vi "Stimulus.Create.vi"(8 "error in (no error)":errorcluster, 11 "State Variables":T1={"Events.State"=refnum, "Events.Test Result"=refnum, "Events.Progress"=refnum, "INI.Settings"={"Build Location"=path "C:/Simple Sequence Editor/SequenceRepo", "LoggingLocation"=path "", "Sequence.AbortChannel"="", "Sequence.IterationInfoChannel"="", "Sequence.DurationChannel"="", "Sequence.StepInfoChannel"="", "Sequence.SkipChannel"="", "PlotChannels"=[], "Sequence.InitializeScript"=path "C:/Simple Sequence Editor/SequenceRepo", "Sequence.CleanupScript"=path "", "Log.DefaultRate"=0.0}, "NIVS.AlarmManager"=refnum, "NIVS.BaseLogPath"=path "", "NIVS.DataLogManagerRef"=refnum, "NIVS.DataLogSpecRef"=refnum, "NIVS.Deployed"=FALSE, "NIVS.Events"={"SequenceEvent"=refnum, "SystemChangeEvent"=refnum, "WorkspaceEvent"=refnum}, "NIVS.GatewayIPAddress"="", "NIVS.DataLogGUID"="", "NIVS.ProfileCallback"=refnum, "NIVS.ProfileRef"=refnum, "NIVS.SequenceState"=enum."Idle", "NIVS.SystemDefinitionFile"=path "", "NIVS.SystemStateRefs"={"CustDatRef"=refnum, "EvtRef"=refnum, "Target State User Event"=refnum}, "NIVS.WorkspaceManager"=refnum, "NIVS.EventLogGUID"="", "NIVS.EventLogManagerRef"=refnum, "NIVS.EventLogSpecRef"=refnum, "NIVS.BaseToolPath"=path "", "Restart.Path"=path "", "Sequence.#ofColumns"=0, "Sequence.Iterations"=0, "Sequence.Channels"=[], "Sequence.ValidConfig?"=FALSE, "Station.ID"="", "UDP.Queue"=refnum, "UI.Abort"=refnum, "UI.Alarms"=refnum, "UI.Apply"=refnum, "UI.Back"=refnum, "UI.BaseFileName"=refnum, "UI.CurrentIteration"=refnum, "UI.CurrentStep"=refnum, "UI.CyclicFrequency"=refnum, "UI.Description"=refnum, "UI.DelayTime"=refnum, "UI.DisableAlarms"=refnum, "UI.Duration"=refnum, "UI.EnableLogging"=refnum, "UI.EnableState"=refnum, "UI.High"=refnum, "UI.LogChannels"=refnum, "UI.Low"=refnum, "UI.MonitoredVariable"=refnum, "UI.Next"=refnum, "UI.NumberOfCycles"=refnum, "UI.OperatorName"=refnum, "UI.Pause"=refnum, "UI.Profile"=refnum, "UI.Revert"=refnum, "UI.Skip"=refnum, "UI.Start"=refnum, "UI.StartIteration"=refnum, "UI.StartStep"=refnum, "UI.TabControl"=refnum, "UI.TotalIterations"=refnum, "UI.WaveformDefinition"=refnum, "UI.WaveformPreview"=refnum, "UI.WorkOrderNumber"=refnum, "UI.Chart"=refnum, "UI.Status"=refnum, "UI.DataView"=refnum, "UI.Table"=refnum, "UI.Multihead"=refnum, "UI.ToolTab"=refnum, "UI.Result"=refnum, "UI.Log Path"=refnum, "UI.ReportPath"=refnum, "UI.RestartPath"=refnum, "UI.AlarmLog"=refnum}) -> (0 "error out":errorcluster, 3 "State Variables":T1={"Events.State"=refnum, "Events.Test Result"=refnum, "Events.Progress"=refnum, "INI.Settings"={"Build Location"=path "C:/Simple Sequence Editor/SequenceRepo", "LoggingLocation"=path "", "Sequence.AbortChannel"="", "Sequence.IterationInfoChannel"="", "Sequence.DurationChannel"="", "Sequence.StepInfoChannel"="", "Sequence.SkipChannel"="", "PlotChannels"=[], "Sequence.InitializeScript"=path "C:/Simple Sequence Editor/SequenceRepo", "Sequence.CleanupScript"=path "", "Log.DefaultRate"=0.0}, "NIVS.AlarmManager"=refnum, "NIVS.BaseLogPath"=path "", "NIVS.DataLogManagerRef"=refnum, "NIVS.DataLogSpecRef"=refnum, "NIVS.Deployed"=FALSE, "NIVS.Events"={"SequenceEvent"=refnum, "SystemChangeEvent"=refnum, "WorkspaceEvent"=refnum}, "NIVS.GatewayIPAddress"="", "NIVS.DataLogGUID"="", "NIVS.ProfileCallback"=refnum, "NIVS.ProfileRef"=refnum, "NIVS.SequenceState"=enum."Idle", "NIVS.SystemDefinitionFile"=path "", "NIVS.SystemStateRefs"={"CustDatRef"=refnum, "EvtRef"=refnum, "Target State User Event"=refnum}, "NIVS.WorkspaceManager"=refnum, "NIVS.EventLogGUID"="", "NIVS.EventLogManagerRef"=refnum, "NIVS.EventLogSpecRef"=refnum, "NIVS.BaseToolPath"=path "", "Restart.Path"=path "", "Sequence.#ofColumns"=0, "Sequence.Iterations"=0, "Sequence.Channels"=[], "Sequence.ValidConfig?"=FALSE, "Station.ID"="", "UDP.Queue"=refnum, "UI.Abort"=refnum, "UI.Alarms"=refnum, "UI.Apply"=refnum, "UI.Back"=refnum, "UI.BaseFileName"=refnum, "UI.CurrentIteration"=refnum, "UI.CurrentStep"=refnum, "UI.CyclicFrequency"=refnum, "UI.Description"=refnum, "UI.DelayTime"=refnum, "UI.DisableAlarms"=refnum, "UI.Duration"=refnum, "UI.EnableLogging"=refnum, "UI.EnableState"=refnum, "UI.High"=refnum, "UI.LogChannels"=refnum, "UI.Low"=refnum, "UI.MonitoredVariable"=refnum, "UI.Next"=refnum, "UI.NumberOfCycles"=refnum, "UI.OperatorName"=refnum, "UI.Pause"=refnum, "UI.Profile"=refnum, "UI.Revert"=refnum, "UI.Skip"=refnum, "UI.Start"=refnum, "UI.StartIteration"=refnum, "UI.StartStep"=refnum, "UI.TabControl"=refnum, "UI.TotalIterations"=refnum, "UI.WaveformDefinition"=refnum, "UI.WaveformPreview"=refnum, "UI.WorkOrderNumber"=refnum, "UI.Chart"=refnum, "UI.Status"=refnum, "UI.DataView"=refnum, "UI.Table"=refnum, "UI.Multihead"=refnum, "UI.ToolTab"=refnum, "UI.Result"=refnum, "UI.Log Path"=refnum, "UI.ReportPath"=refnum, "UI.RestartPath"=refnum, "UI.AlarmLog"=refnum})   [LabVIEW 2015, in "Single Station Execution.lvlib"]
uses:
  Single Station Execution.lvlib
  Types/Main.StateVariables.ctl
  Types/INI.Settings.ctl
  <vilib>/NI Veristand/Execution/AlarmManager/AlarmManagerAPI.ctl
  NationalInstruments.VeriStand.ClientAPI
  <vilib>/NI Veristand/Execution/DataLogging/IDataLogging Ref.ctl
  <vilib>/NI Veristand/Execution/DataLogging/DataLoggingSpecification Ref.ctl
  Types/Execute.UserEventRefs.ctl
  <vilib>/NI Veristand/Execution/Workspace/SystemStateRegEventRef.ctl
  <vilib>/NI Veristand/Execution/Workspace/Target State Info.ctl
  <vilib>/NI Veristand/Execution/Workspace/Target State.ctl
  NationalInstruments.VeriStand.RealTimeSequenceDefinitionApi
  Types/Execution.SequenceState.ctl
  <vilib>/NI Veristand/Execution/Workspace/SystemStateEventRef.ctl
  <vilib>/NI Veristand/Execution/Workspace/WorkspaceAPI.ctl
  Types/UDPEngine.QueueCluster.ctl
  Types/UDPEngine.State.ctl
  Types/Restart.Settings.ctl
  <vilib>/NI Veristand/Execution/DataLogging/TDMS Channel Group.ctl
  <vilib>/NI Veristand/Execution/DataLogging/TDMS Property.ctl
  <vilib>/NI Veristand/Execution/DataLogging/TDMS Channel.ctl
  <vilib>/NI Veristand/Execution/DataLogging/Time Channel Options.ctl
  Types/Log.SelectedChannels.ctl
  Types/Config.AlarmSettings.ctl
  Types/Compiled.RTSequenceProperties.ctl
  Types/Channel.Properties.ctl
  Types/Compiled.StepProperties.ctl
  Types/Compiled.IOStateProperties.ctl
  Types/Compiled.StepElementProperties.ctl
  Types/Step.Types.ctl
  Types/Compiled.StepCondition.ctl
  Types/Conditions.OperationTypes.ctl
  Types/Compiled.SequenceChannels.ctl
  NationalInstruments.VeriStand.DataTypes
  NationalInstruments.VeriStand
  <vilib>/NI Veristand/Execution/DataLogging/File Conflict Operation.ctl
  <vilib>/NI Veristand/Execution/DataLogging/Slope.ctl
  Main.Constants.vi
  <vilib>/NI Veristand/Execution/DataLogging/New Data Logging Specification (TDMS).vi
  <vilib>/NI Veristand/Execution/DataLogging/Set Data Logging Rate (Target Rate).vi
  <vilib>/NI Veristand/Execution/DataLogging/Set Data Logging Rate (Custom Rate).vi
  <vilib>/NI Veristand/Execution/DataLogging/Set Start Trigger (Start Immediately).vi
  <vilib>/NI Veristand/Execution/DataLogging/Set Start Trigger (Digital Edge).vi
  <vilib>/NI Veristand/Execution/DataLogging/Set Stop Trigger (Duration).vi
  <vilib>/NI Veristand/Execution/DataLogging/NI_VS Data Logging API.lvlib
  <vilib>/NI Veristand/Execution/Workspace/NI_VS Workspace ExecutionAPI.lvlib
  <vilib>/NI Veristand/Execution/AlarmManager/NI_VS AlarmManager ExecutionAPI.lvlib
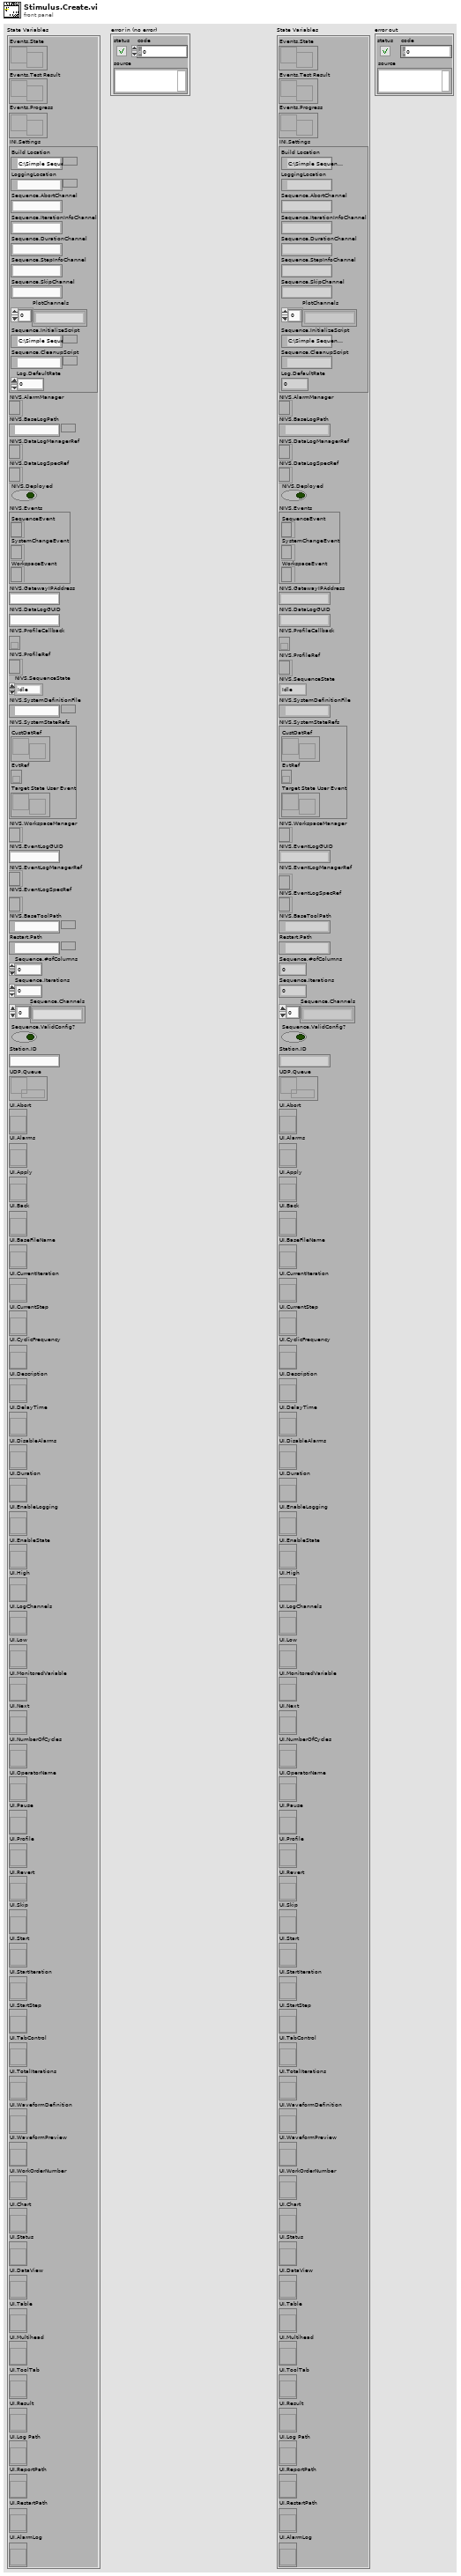
[diagram p1: front panel]
types:
  T1 = typedef "Single Station Execution.lvlib/Main.StateVariables.ctl" = cluster{"Events.State":refnum<user-event>, "Events.Test Result":refnum<user-event>, "Events.Progress":refnum<user-event>, "INI.Settings":T2, "NIVS.AlarmManager":T3, "NIVS.BaseLogPath":path, "NIVS.DataLogManagerRef":T4, "NIVS.DataLogSpecRef":T5, "NIVS.Deployed":bool, "NIVS.Events":T6, "NIVS.GatewayIPAddress":string, "NIVS.DataLogGUID":string, "NIVS.ProfileCallback":refnum<k27>, "NIVS.ProfileRef":refnum<k24>, "NIVS.SequenceState":T8, "NIVS.SystemDefinitionFile":path, "NIVS.SystemStateRefs":T9, "NIVS.WorkspaceManager":T10, "NIVS.EventLogGUID":string, "NIVS.EventLogManagerRef":T4, "NIVS.EventLogSpecRef":T5, "NIVS.BaseToolPath":path, "Restart.Path":path, "Sequence.#ofColumns":i32, "Sequence.Iterations":u32, "Sequence.Channels":string[], "Sequence.ValidConfig?":bool, "Station.ID":string, "UDP.Queue":refnum<queue>, "UI.Abort":refnum<vi>, "UI.Alarms":refnum<vi>, "UI.Apply":refnum<vi>, "UI.Back":refnum<vi>, "UI.BaseFileName":refnum<vi>, "UI.CurrentIteration":refnum<vi>, "UI.CurrentStep":refnum<vi>, "UI.CyclicFrequency":refnum<vi>, "UI.Description":refnum<vi>, "UI.DelayTime":refnum<vi>, "UI.DisableAlarms":refnum<vi>, "UI.Duration":refnum<vi>, "UI.EnableLogging":refnum<vi>, "UI.EnableState":refnum<vi>, "UI.High":refnum<vi>, "UI.LogChannels":refnum<vi>, "UI.Low":refnum<vi>, "UI.MonitoredVariable":refnum<vi>, "UI.Next":refnum<vi>, "UI.NumberOfCycles":refnum<vi>, "UI.OperatorName":refnum<vi>, "UI.Pause":refnum<vi>, "UI.Profile":refnum<vi>, "UI.Revert":refnum<vi>, "UI.Skip":refnum<vi>, "UI.Start":refnum<vi>, "UI.StartIteration":refnum<vi>, "UI.StartStep":refnum<vi>, "UI.TabControl":refnum<vi>, "UI.TotalIterations":refnum<vi>, "UI.WaveformDefinition":refnum<vi>, "UI.WaveformPreview":refnum<vi>, "UI.WorkOrderNumber":refnum<vi>, "UI.Chart":refnum<vi>, "UI.Status":refnum<vi>, "UI.DataView":refnum<vi>, "UI.Table":refnum<vi>, "UI.Multihead":refnum<vi>, "UI.ToolTab":refnum<vi>, "UI.Result":refnum<vi>, "UI.Log Path":refnum<vi>, "UI.ReportPath":refnum<vi>, "UI.RestartPath":refnum<vi>, "UI.AlarmLog":refnum<vi>}
  T2 = typedef "Single Station Execution.lvlib/INI.Settings.ctl" = cluster{"Build Location":path, "LoggingLocation":path, "Sequence.AbortChannel":string, "Sequence.IterationInfoChannel":string, "Sequence.DurationChannel":string, "Sequence.StepInfoChannel":string, "Sequence.SkipChannel":string, "PlotChannels":string[], "Sequence.InitializeScript":path, "Sequence.CleanupScript":path, "Log.DefaultRate":dbl}
  T3 = typedef "NI_VS AlarmManager ExecutionAPI.lvlib/AlarmManagerAPI.ctl" = refnum<k24>
  T4 = typedef "NI_VS Data Logging API.lvlib/IDataLogging Ref.ctl" = refnum<k24>
  T5 = typedef "NI_VS Data Logging API.lvlib/DataLoggingSpecification Ref.ctl" = refnum<k24>
  T6 = typedef "Single Station Execution.lvlib/Execute.UserEventRefs.ctl" = cluster{"SequenceEvent":refnum<event-registration>, "SystemChangeEvent":T7, "WorkspaceEvent":refnum<event-registration>}
  T7 = typedef "NI_VS Workspace ExecutionAPI.lvlib/SystemStateRegEventRef.ctl" = refnum<event-registration>
  T8 = typedef "Single Station Execution.lvlib/Execution.SequenceState.ctl" = enum16{"Idle", "Initializing", "Running", "Paused", "Finalizing", "Complete"}
  T9 = typedef "NI_VS Workspace ExecutionAPI.lvlib/SystemStateEventRef.ctl" = cluster{"CustDatRef":refnum<user-event>, "EvtRef":refnum<k27>, "Target State User Event":refnum<user-event>}
  T10 = typedef "NI_VS Workspace ExecutionAPI.lvlib/WorkspaceAPI.ctl" = refnum<k24>
  T11 = typedef "Single Station Execution.lvlib/Compiled.StepProperties.ctl" = cluster{"IOState":T12, "Condition":T16}
  T12 = typedef "Single Station Execution.lvlib/Compiled.IOStateProperties.ctl" = cluster{"Duration":dbl, "Elements":T13[]}
  T13 = typedef "Single Station Execution.lvlib/Compiled.StepElementProperties.ctl" = cluster{"Channel":T14, "Step":T15, "Parameters":dbl[]}
  T14 = typedef "Single Station Execution.lvlib/Channel.Properties.ctl" = cluster{"Name":string, "NodePath":string, "ScaleUnits":string}
  T15 = typedef "Single Station Execution.lvlib/Step.Types.ctl" = enum8{"Step", "iStep", "Ramp", "Unchanged", "Unknown", "Sine", "LogSine", "LinearSine", "ForcedRamp", "Waveform"}
  T16 = typedef "Single Station Execution.lvlib/Compiled.StepCondition.ctl" = cluster{"First Opreation":T17, "Expression":string}
  T17 = typedef "Single Station Execution.lvlib/Conditions.OperationTypes.ctl" = enum8{"None", "&&", "||"}
  T18 = typedef "Single Station Execution.lvlib/Compiled.RTSequenceProperties.ctl" = cluster{"Channels":T14[], "Steps":T11[], "Iterations":u32, "Sequence Channels":T19}
  T19 = typedef "Single Station Execution.lvlib/Compiled.SequenceChannels.ctl" = cluster{"Abort":T14, "IterationInfo":T14, "StepInfo":T14, "Skip":T14, "Duration":T14}
  T20 = typedef "Single Station Execution.lvlib/Restart.Settings.ctl" = cluster{"LogFile":path, "Log Settings":T21[], "StimulusProfile":path, "StopIteration":u32, "StopStep":u32, "Log Channels":T25, "Base File Name":string, "Enable Logging":bool, "Profile":string, "StopDuration":dbl, "Waveform Definition":path, "Number of Cycles":dbl, "Cyclic Frequency":dbl, "Work Order Number":string, "Operator Name":string, "Description":string, "Station.ID":string, "Sequence.Channels":string[], "Alarms":T26[]}
  T21 = typedef "NI_VS Data Logging API.lvlib/TDMS Channel Group.ctl" = cluster{"Group Name":string, "Group Description":string, "Group Properties":T22[], "Channels":T23[], "Time Channel Options":T24, "Time Channel Name":string}
  T22 = typedef "NI_VS Data Logging API.lvlib/TDMS Property.ctl" = cluster{"Name":string, "Value":variant}
  T23 = typedef "NI_VS Data Logging API.lvlib/TDMS Channel.ctl" = cluster{"Channel Name":string, "Channel Path":string, "Channel Description":string, "Channel Properties":T22[]}
  T24 = typedef "NI_VS Data Logging API.lvlib/Time Channel Options.ctl" = enum16{"No Time Channel", "Absolute Time", "System Time", "System Time - Microseconds", "Absolute Time as Double"}
  T25 = typedef "Single Station Execution.lvlib/Log.SelectedChannels.ctl" = enum16{"Channels (No System Channel)", "Aliases", "All"}
  T26 = typedef "Single Station Execution.lvlib/Config.AlarmSettings.ctl" = cluster{"Watch Channel":string, "High Limit":dbl, "Low Limit":dbl, "Delay":dbl, "State":enum16{"Disabled", "Enabled", "Tripped", "Delayed Trip", "Indicate"}, "Alarm Name":string}
  T27 = typedef "Single Station Execution.lvlib/Saved.Sequence.ctl" = cluster{"Output Channels":T14[], "Data":dbl[][]}
  T28 = cluster{"Channels[0]":T14, "Channels[1]":T14, "Channels[2]":T14, "Channels[3]":T14, "Channels[4]":T14}
  T29 = enum16{"Channels (No System Channel)", "Aliases", "All"}
  T30 = typedef "NI_VS Data Logging API.lvlib/File Conflict Operation.ctl" = enum16{"Create Unique", "Append to Existing", "Overwrite"}
  T31 = typedef "NI_VS Data Logging API.lvlib/Slope.ctl" = enum16{"Rising", "Falling"}
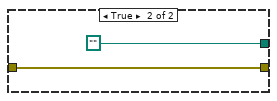
[diagram p5: hidden frame]
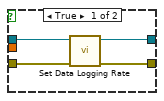
[diagram p7: hidden frame]
diagram:
  w90 = "_" ("string")
  w128 = u32 0 ("minor")
  n1 = Unbundle By Name("State Variables") -> ("INI.Settings.Log.DefaultRate"=w21:dbl, "UI.Log Path"=w22:refnum<vi>, "NIVS.WorkspaceManager"=w15:T10, "UI.EnableLogging"=w142:refnum<vi>, "UI.LogChannels"=w138:refnum<vi>, "UI.BaseFileName"=w139:refnum<vi>, "UI.StartStep"=w148:refnum<vi>, "UI.StartIteration"=w150:refnum<vi>, "UI.Profile"=w94:refnum<vi>, "INI.Settings.Sequence.AbortChannel"=w12:string, "INI.Settings.Sequence.IterationInfoChannel"=w117:string, "INI.Settings.Sequence.StepInfoChannel"=w116:string, "INI.Settings.Sequence.SkipChannel"=w115:string, "INI.Settings.Sequence.DurationChannel"=w114:string, "INI.Settings.Sequence.InitializeScript"=w33:path, "INI.Settings.Sequence.CleanupScript"=w31:path, "NIVS.BaseLogPath"=w34:path, "Station.ID"=w1:string, "UI.WaveformDefinition"=w72:refnum<vi>, "UI.TotalIterations"=w5:refnum<vi>, "UI.NumberOfCycles"=w71:refnum<vi>, "UI.CyclicFrequency"=w70:refnum<vi>, "UI.WorkOrderNumber"=w92:refnum<vi>, "UI.OperatorName"=w93:refnum<vi>, "UI.Description"=w66:refnum<vi>, "UI.Alarms"=w9:refnum<vi>)
  n2 = call "Alarms.CacheCurrentValues.vi"("Station.ID"=w1, "error in (no error)"="error in (no error)", "ListBox in"=w9) -> ("error out"=w7:errorcluster, "Alarms"=w6:T26[])  [unwired: 7 in]
  n3 = property class="Str"(reference=w66, error in=w7) -> (error out=w67:errorcluster, "Value"=w85:string)  [unwired: 1 out]
  n4 = property class="Str"(reference=w93, error in=w67) -> (error out=w68:errorcluster, "Value"=w86:string)  [unwired: 1 out]
  n5 = property class="Str"(reference=w92, error in=w68) -> (error out=w69:errorcluster, "Value"=w87:string)  [unwired: 1 out]
  n6 = property class="DigNum (strict)"(reference=w70, error in=w69) -> (error out=w109:errorcluster, "Value"=w88:dbl)  [unwired: 1 out]
  n7 = Reciprocal(x=w88) -> (1/x=w107:dbl)
  n8 = property class="DigNum (strict)"(reference=w71, error in=w109) -> (error out=w3:errorcluster, "Value"=w4:u32)  [unwired: 1 out]
  n9 = property class="DigNum (strict)"(reference=w5, error in=w3, "Value"=w4) -> (error out=w2:errorcluster)  [unwired: 1 out]
  n10 = property class="Path"(reference=w72, error in=w2) -> (error out=w62:errorcluster, "Value"=w89:path)  [unwired: 1 out]
  n11 = Empty String/Path?(string/path=w116) -> (empty?=w126:bool)
  n12 = call <vilib>:"Get File Extension.vi"("error in (no error)"=w62, "file"=w89) -> ("error out"=w65:errorcluster, "filename without extension"=w95:string, "dup file"=w99:path)  [unwired: 5 in, 2 out]
  n13 = call "Log.CreateTimeInfo.vi"() -> ("String"=w134:string, "File Folder"=w135:path)  [unwired: 10 in]
  n14 = Empty String/Path?(string/path=w117) -> (empty?=w127:bool)
  n15 = Build Array(w12, w117, w116, w115, w114) -> (w113:string[])
  n16 = Build Path(base path=w34, name or relative path=w135) -> (appended path=w100:path)
  n17 = Compound Arithmetic op=OR(w126, w127) -> (w101:bool)
  n18 = call "App.OpenWaveformDefinition.vi"("StationID"=w1, "error in (no error)"=w65, "selected path"=w99) -> ("error out"=w61:errorcluster, "Settings"=w118:T27)  [unwired: 7 in]
  n19 = Concatenate Strings(w1, w90, w95, ".nivsstimprof" ("string")) -> (w57:string)
  n20 = Concatenate Strings(w1, w90, w95, ".nivsseq" ("string")) -> (w97:string)
  n21 = Create Folder(path (use dialog)=w100, error in=w61) -> (created path=w20:path, error out=w25:errorcluster)  [unwired: 1 in, 1 out]
  n22 = Build Path(base path=w20, name or relative path="Test Files") -> (appended path=w26:path)
  n23 = Create Folder(path (use dialog)=w26, error in=w25) -> (created path=w23:path, error out=w24:errorcluster)  [unwired: 1 in, 1 out]
  n24 = Build Path(base path=w23, name or relative path=w57) -> (appended path=w84:path)
  n25 = Build Path(base path=w23, name or relative path=w97) -> (appended path=w83:path)
  n26 = call "File.Copy.vi"("error in (no error)"=w24, "Copy Directory"=w23, "Source File"=w31) -> ("error out"=w32:errorcluster, "NewPath"=w29:path)  [unwired: 7 in]
  n27 = call "File.Copy.vi"("error in (no error)"=w32, "Copy Directory"=w23, "Source File"=w33) -> ("error out"=w30:errorcluster, "NewPath"=w28:path)  [unwired: 7 in]
  n28 = call "Channels.Format.vi"("error in (no error)"=w30, "Channels"=w113) -> ("error out"=w59:errorcluster, "Channels"=w91:T14[], "Channels (no blanks)"=w112:T14[])  [unwired: 7 in]
  n29 = Unbundle By Name(w118) -> ("Output Channels"=w106:T14[], "Data"=w105:dbl[][])
  n30 = Array To Cluster(array=w91) -> (cluster=w60:T28)
  n31 = for {
    tunnel: w106 -> [w168] mode=indexing
    tunnel: w105 -> [w171]
    tunnel: [w166] -> w104 mode=indexing
    i -> [w170]
    n32 = Index Array(array=w171, index (col)=w170) -> (element=w167:dbl[])  [unwired: 1 in]
    n33 = Bundle By Name(cluster=T13 {"Channel"={"Name"="", "NodePath"="", "ScaleUnits"=""}, "Step"=enum."Waveform", "Parameters"=[]}, "Channel"=w168, "Parameters"=w167) -> (w166:T13)
  }
  n34 = Build Array (concatenate)(w112, w106) -> (w58:T14[])
  n35 = for {
    tunnel: w106 -> [w173] mode=indexing
    tunnel: [w172] -> w45 mode=indexing
    n36 = Unbundle By Name(w173) -> ("NodePath"=w172:string)
  }
  n37 = To Variant(anything=w1) -> (Variant=w82:variant)
  n38 = To Variant(anything=w84) -> (Variant=w81:variant)
  n39 = To Variant(anything=w89) -> (Variant=w80:variant)
  n40 = To Variant(anything=w4) -> (Variant=w79:variant)
  n41 = To Variant(anything=w88) -> (Variant=w78:variant)
  n42 = To Variant(anything=w87) -> (Variant=w77:variant)
  n43 = To Variant(anything=w86) -> (Variant=w76:variant)
  n44 = To Variant(anything=w85) -> (Variant=w75:variant)
  n45 = Strip Path(path=w84) -> (name=w64:string)  [unwired: 1 out]
  n46 = Build Array(w82, w81, w80, w79, w78, w77, w76, w75) -> (w74:variant[])
  n47 = for {
    tunnel: w74 -> [w177] mode=indexing
    tunnel: string[] ["StationID", "StimulusProfile", "WaveformDefinition", "NumberOfCycles", "CyclicFrequency", "WorkOrderNumber", "Operator", "Description"] -> [w175] mode=indexing
    tunnel: [w174] -> w13 mode=indexing
    n48 = Bundle By Name(cluster=T22 {"Name"="", "Value"=variant} ("TDMS Property"), "Value"=w177, "Name"=w175) -> (w174:T22)
  }
  n49 = Bundle By Name(cluster=T11 {"IOState"={"Duration"=0.0, "Elements"=[]}, "Condition"={"First Opreation"=enum."None", "Expression"=""}} ("Step"), "IOState.Elements"=w104, "IOState.Duration"=w107) -> (w103:T11)
  n50 = Bundle By Name(cluster=T20 {"LogFile"=path "", "Log Settings"=[], "StimulusProfile"=path "", "StopIteration"=0, "StopStep"=0, "Log Channels"=enum."Aliases", "Base File Name"="Log", "Enable Logging"=TRUE, "Profile"="", "StopDuration"=0.0, "Waveform Definition"=path "", "Number of Cycles"=0.0, "Cyclic Frequency"=0.0, "Work Order Number"="", "Operator Name"="", "Description"="", "Station.ID"="", "Sequence.Channels"=[], "Alarms"=[]}, "Sequence.Channels"=w45, "Station.ID"=w1, "Waveform Definition"=w89, "Number of Cycles"=w4, "Cyclic Frequency"=w88, "Work Order Number"=w87, "Operator Name"=w86, "Description"=w85, "StimulusProfile"=w84, "Profile"=w64, "Alarms"=w6) -> (w124:T20)
  n51 = Build Array(w103) -> (w102:T11[])
  n52 = Bundle By Name(cluster=T18 {"Channels"=[], "Steps"=[], "Iterations"=0, "Sequence Channels"={"Abort"={"Name"="", "NodePath"="", "ScaleUnits"=""}, "IterationInfo"={"Name"="", "NodePath"="", "ScaleUnits"=""}, "StepInfo"={"Name"="", "NodePath"="", "ScaleUnits"=""}, "Skip"={"Name"="", "NodePath"="", "ScaleUnits"=""}, "Duration"={"Name"="", "NodePath"="", "ScaleUnits"=""}}} ("Compiled Settings"), "Channels"=w58, "Sequence Channels"=w60, "Iterations"=w4, "Steps"=w102) -> (w110:T18)
  n53 = call "Sequence.GenerateSequence.vi"("error in (no error)"=w59, "Compiled Settings"=w110, "Path"=w83) -> ("error out"=w63:errorcluster)  [unwired: 8 in]
  n54 = property class="Str"(reference=w94, error in=w63, "Value"=w57) -> (error out=w50:errorcluster)  [unwired: 1 out]
  n55 = Path To String(path=w83) -> (string=w163:string)
  n56 = constructor class="RealTimeSequenceCallStep"(error in=w50, "sequencePath"=w163) -> (reference out=w152:refnum<k24>, error out=w54:errorcluster)  [unwired: 2 in, 2 out]
  n57 = property class="DigNum (strict)"(reference=w150, error in=w54) -> (error out=w149:errorcluster, "Value"=w133:u32)  [unwired: 1 out]
  n58 = global read "Main.Constants.vi" "Sequence.StartingIteration"() -> (w145:string)
  n59 = global read "Main.Constants.vi" "Sequence.StartingStep"() -> (w146:string)
  n60 = property class="DigNum (strict)"(reference=w148, error in=w149) -> (error out=w49:errorcluster, "Value"=w56:u32)  [unwired: 1 out]
  n61 = Build Array(w56, w133) -> (w147:u32[])
  n62 = Build Array(w146, w145) -> (w144:string[])
  n63 = for {
    tunnel: w144 -> [w180] mode=indexing
    tunnel: w147 -> [w178] mode=indexing
    shift-right: [w185] -> w151
    shift-left: w152 -> [w186]
    shift-right: [w187] -> w153
    shift-left: w49 -> [w181]
    n64 = constructor class="U32Value"(error in=w181, "Value"=w178) -> (reference out=w183:refnum<k24>, error out=w182:errorcluster)  [unwired: 2 in, 2 out]
    n65 = constructor class="RealTimeSequenceCallParameterAs"(error in=w182, "parameterName"=w180, "value"=w183) -> (reference out=w184:refnum<k24>, error out=w179:errorcluster)  [unwired: 2 in, 3 out]
    n66 = invoke class="RealTimeSequenceCallStep" method="AddReplaceParameterAssignment"(reference=w186, error in=w179, "parameterAssignment"=w184) -> (reference out=w185:refnum<k24>, error out=w187:errorcluster)  [unwired: 1 in, 2 out]
  }
  n67 = constructor class="StimulusProfile"(error in=w153) -> (reference out=w42:refnum<k24>, error out=w44:errorcluster)  [unwired: 2 in, 1 out]
  n68 = Build Array(w151) -> (w161:refnum<k24>[])
  n69 = Empty String/Path?(string/path=w28) -> (empty?=w40:bool)
  n70 = case shown="False" w40 {
    tunnel: w44 -> [w198 w201]
    tunnel: [w196 w201] -> w43
    tunnel: w42 -> [w195 w200]
    tunnel: [w194 w200] -> w41
    tunnel: w28 -> [w193 _]
    tunnel: w1 -> [w188 _]
    frame False {
      n71 = Path To String(path=w193) -> (string=w199:string)
      n72 = constructor class="RealTimeSequenceCallStep"(error in=w198, "sequencePath"=w199) -> (reference out=w190:refnum<k24>, error out=w192:errorcluster)  [unwired: 2 in, 2 out]
      n73 = call "Sequence.Parameterize.vi"("error in (no error)"=w192, "Station.ID"=w188, "Sequence"=w190) -> ("error out"=w191:errorcluster, "Sequence"=w189:refnum<k24>)  [unwired: 7 in]
      n74 = Build Array(w189) -> (w197:refnum<k24>[])
      n75 = property class="StimulusProfile"(reference=w195, error in=w191, "Setup.Steps"=w197) -> (reference out=w194:refnum<k24>, error out=w196:errorcluster)
    }
    frame True {
    }
  }
  n76 = Path To String(path=w20) -> (string=w132:string)
  n77 = property class="StimulusProfile"(reference=w41, error in=w43, "Main.Steps"=w161, "ResultsDirectory"=w132) -> (reference out=w36:refnum<k24>, error out=w38:errorcluster)
  n78 = Empty String/Path?(string/path=w29) -> (empty?=w39:bool)
  n79 = case shown="False" w39 {
    tunnel: w38 -> [w212 w215]
    tunnel: [w210 w215] -> w37
    tunnel: w36 -> [w209 w214]
    tunnel: [w208 w214] -> w35
    tunnel: w29 -> [w207 _]
    tunnel: w1 -> [w202 _]
    frame False {
      n80 = Path To String(path=w207) -> (string=w213:string)
      n81 = constructor class="RealTimeSequenceCallStep"(error in=w212, "sequencePath"=w213) -> (reference out=w206:refnum<k24>, error out=w204:errorcluster)  [unwired: 2 in, 2 out]
      n82 = call "Sequence.Parameterize.vi"("error in (no error)"=w204, "Station.ID"=w202, "Sequence"=w206) -> ("error out"=w203:errorcluster, "Sequence"=w205:refnum<k24>)  [unwired: 7 in]
      n83 = Build Array(w205) -> (w211:refnum<k24>[])
      n84 = property class="StimulusProfile"(reference=w209, error in=w203, "CleanUp.Steps"=w211) -> (reference out=w208:refnum<k24>, error out=w210:errorcluster)
    }
    frame True {
    }
  }
  n85 = call "Sequence.GetVersion.vi"("error in (no error)"=w37, "Exists"=TRUE, "Path"=w83) -> ("error out"=w55:errorcluster, "Build"=w130:u32)  [unwired: 7 in]
  n86 = constructor class="XMLVersionInfo"(error in=w55, "major"=u32 1, "minor"=w128, "fix"=w128, "build"=w130) -> (reference out=w53:refnum<k24>, error out=w52:errorcluster)  [unwired: 2 in, 5 out]
  n87 = property class="StimulusProfile"(reference=w35, error in=w52, "Version"=w53) -> (reference out=w47:refnum<k24>, error out=w51:errorcluster)
  n88 = Path To String(path=w84) -> (string=w162:string)
  n89 = invoke class="StimulusProfile" method="SaveStimulusProfile"(reference=w47, error in=w51, "file"=w162) -> (reference out=w159:refnum<k24>, error out=w158:errorcluster)  [unwired: 1 in, 2 out]
  n90 = invoke class="StimulusProfile" method="CheckForErrors"(reference=w159, error in=w158) -> (reference out=w136:refnum<k24>, error out=w156:errorcluster, "CheckForErrors"=w157:refnum<k24>[])  [unwired: 1 in]
  n91 = for {
    tunnel: w157 -> [w222] mode=indexing
    tunnel: [w217] -> w154 mode=indexing
    shift-right: [w216] -> w155
    shift-left: w156 -> [w221]
    n92 = property class="CompilationEvent"(reference=w222, error in=w221) -> (error out=w216:errorcluster, "Code"=w219:i32, "SourceFile"=w218:string)  [unwired: 1 out]
    n93 = Bundle By Name(cluster=errorcluster {"status"=TRUE, "code"=0, "source"=""} ("error out"), "code"=w219, "source"=w218) -> (w217:errorcluster)
  }
  n94 = Merge Errors(w155, w154) -> (w137:errorcluster)
  n95 = property class="Str"(reference=w139, error in=w137) -> (error out=w160:errorcluster, "Value"=w46:string)  [unwired: 1 out]
  n96 = property class="Enum (strict)"(reference=w138, error in=w160) -> (error out=w140:errorcluster, "Value"=w16:T29)  [unwired: 1 out]
  n97 = property class="Bool (strict)"(reference=w142, error in=w140) -> (error out=w141:errorcluster, "Value"=w48:bool)  [unwired: 1 out]
  n98 = Bundle By Name(cluster=w124, "Enable Logging"=w48, "Log Channels"=w16, "Base File Name"=w46) -> (w123:T20)
  n99 = case shown="True" w48 {
    tunnel: w141 -> [w225 w252]
    tunnel: [w225 w244] -> w17
    tunnel: w46 -> [_ w237]
    tunnel: w16 -> [_ w250]
    tunnel: w15 -> [_ w251]
    tunnel: [_ w243] -> w143
    tunnel: w20 -> [w223 w226]
    tunnel: w134 -> [_ w239]
    tunnel: w123 -> [w224 w227]
    tunnel: [w224 w236] -> w121
    tunnel: [w223 w226] -> w120
    tunnel: w13 -> [_ w235]
    tunnel: w1 -> [_ w234]
    tunnel: w22 -> [_ w231]
    tunnel: w21 -> [_ w228]
    frame False {
    }
    frame True {
      n100 = call "Log.CreateChannelList.vi"("error in (no error)"=w252, "Station.ID"=w234, "Value"=w250, "Workspace"=w251) -> ("error out"=w233:errorcluster, "Channel List"=w238:T21[])  [unwired: 6 in]
      n101 = Concatenate Strings(w237, "_" ("string"), w239, ".tdms" ("string")) -> (w241:string)
      n102 = Build Path(base path=w226, name or relative path=w241) -> (appended path=w230:path)
      n103 = property class="Path"(reference=w231, error in=w233, "Value"=w226) -> (error out=w232:errorcluster)  [unwired: 1 out]
      n104 = call-poly <vilib>:"New Data Logging Specification.vi"("File Properties"=w235, "error in (no error)"=w232, "Channel Groups"=w238, "File Conflict Operation"=File_Conflict_Operation."Create Unique", "Base Log File Path"=w230) -> ("error out"=w246:errorcluster, "Data Logging Specification Ref out"=w249:T5)  [unwired: 5 in]
      n105 = Less Than 0?(x=w228) -> (x < 0?=w229:bool)
      n106 = Bundle By Name(cluster=w227, "LogFile"=w230, "Log Settings"=w238) -> (w236:T20)
      n107 = case shown="False" w229 {
        tunnel: w249 -> [w256 w261]
        tunnel: [w255 w260] -> w248
        tunnel: [w254 w259] -> w247
        tunnel: w246 -> [w253 w258]
        tunnel: w228 -> [_ w257]
        frame True {
          n108 = call-poly <vilib>:"Set Data Logging Rate.vi"("error in (no error)"=w253, "Data Logging Specification Ref in"=w256) -> ("error out"=w254:errorcluster, "Data Logging Specification Ref out"=w255:T5)  [unwired: 8 in]
        }
        frame False {
          n109 = call-poly <vilib>:"Set Data Logging Rate.vi"("error in (no error)"=w258, "Custom Rate (Hz)"=w257, "Data Logging Specification Ref in"=w261) -> ("error out"=w259:errorcluster, "Data Logging Specification Ref out"=w260:T5)  [unwired: 7 in]
        }
      }
      n110 = call-poly <vilib>:"Set Start Trigger.vi"("error in (no error)"=w247, "Data Logging Specification Ref in"=w248) -> ("error out"=w244:errorcluster, "Data Logging Specification Ref out"=w243:T5)  [unwired: 8 in]
    }
  }
  n111 = Build Path(base path=w20, name or relative path="CrashLog {Month} {Day} {Year} {Hour} {Minute} {Second}.tdms") -> (appended path=w14:path)
  n112 = Empty String/Path?(string/path=w12) -> (empty?=w18:bool)
  n113 = case shown="False" w18 {
    tunnel: w17 -> [w283 w284]
    tunnel: [w269 w284] -> w10
    tunnel: w12 -> [w276 _]
    tunnel: [w268 _] -> w11
    tunnel: w13 -> [w271 _]
    tunnel: w15 -> [w265 _]
    tunnel: w16 -> [w264 _]
    tunnel: w1 -> [w263 _]
    tunnel: w14 -> [w262 _]
    frame False {
      n114 = call "Log.CreateChannelList.vi"("error in (no error)"=w283, "Station.ID"=w263, "Value"=w264, "Workspace"=w265) -> ("error out"=w277:errorcluster, "Channel List"=w272:T21[])  [unwired: 6 in]
      n115 = call-poly <vilib>:"New Data Logging Specification.vi"("File Properties"=w271, "error in (no error)"=w277, "Channel Groups"=w272, "File Conflict Operation"=File_Conflict_Operation."Create Unique", "Base Log File Path"=w262) -> ("error out"=w281:errorcluster, "Data Logging Specification Ref out"=w278:T5)  [unwired: 5 in]
      n116 = call-poly <vilib>:"Set Data Logging Rate.vi"("error in (no error)"=w281, "Data Logging Specification Ref in"=w278) -> ("error out"=w280:errorcluster, "Data Logging Specification Ref out"=w279:T5)  [unwired: 8 in]
      n117 = call-poly <vilib>:"Set Start Trigger.vi"("Retriggerable (F)"=FALSE, "Pre-Trigger Duration (0 s)"=60.0, "error in (no error)"=w280, "Trigger Channel"=w276, "Slope"=Slope."Rising", "Data Logging Specification Ref in"=w279) -> ("error out"=w270:errorcluster, "Data Logging Specification Ref out"=w267:T5)  [unwired: 4 in]
      n118 = call-poly <vilib>:"Set Stop Trigger.vi"("error in (no error)"=w270, "Duration"=1.0, "Data Logging Specification Ref in"=w267) -> ("error out"=w269:errorcluster, "Data Logging Specification Ref out"=w268:T5)  [unwired: 7 in]
    }
    frame True {
    }
  }
  n119 = case shown="False" w101 {
    tunnel: [w292 w295] -> w122
    tunnel: w10 -> [w293 w295]
    tunnel: w121 -> [w291 _]
    tunnel: w120 -> [w290 _]
    tunnel: [w288 path ""] -> w119
    tunnel: w1 -> [w285 _]
    frame False {
      n120 = Concatenate Strings(w285, "_Restart.info" ("name or relative path")) -> (w286:string)
      n121 = Build Path(base path=w290, name or relative path=w286) -> (appended path=w289:path)
      n122 = call "Restart.SaveSettings.vi"("error in"=w293, "Restart Settings"=w291, "datalog path (use dialog)"=w289) -> ("error out"=w292:errorcluster, "path"=w288:path)  [unwired: 7 in]
    }
    frame True {
    }
  }
  "error out" <- w122
  n123 = Bundle By Name(cluster="State Variables", "Restart.Path"=w119, "NIVS.EventLogSpecRef"=w11, "NIVS.DataLogSpecRef"=w143, "NIVS.ProfileRef"=w136, "Sequence.Channels"=w45) -> (→"State Variables":T1)
